vi "TLPM Measure Power2.vi"(8 "error in (no error)":errorcluster {"code" format="%.0x"}, 11 "instrument handle":refnum<visa-resource-name>) -> (0 "error out":errorcluster {"code" format="%.0x"}, 2 "Power":dbl, 3 "instrument handle out":refnum<visa-resource-name>)   [LabVIEW 2023, in "Thorlabs Power Meter.lvlib"]
doc: "This VI is used to obtain power readings from the instrument. \n\nRemark:\nThis VI starts a new measurement cycle and after finishing measurement the result is received. Subject to the actual Average Count this may take up to seconds. Refer to <Set/Get Average Count>."
uses:
  Thorlabs Power Meter.lvlib
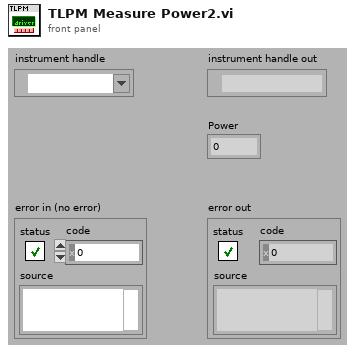
[diagram p1: front panel]
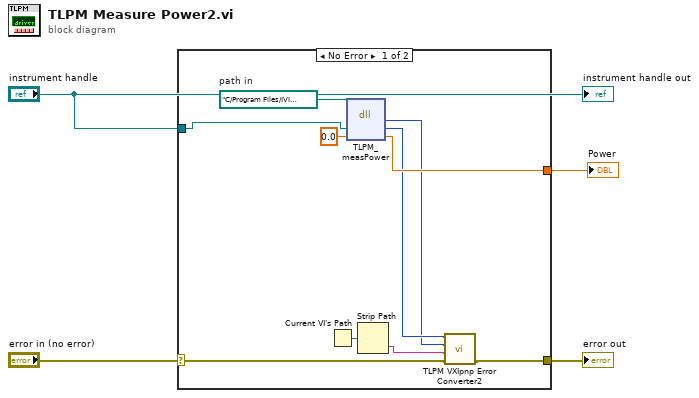
[diagram p0: block diagram]
diagram:
  n1 = case shown="No Error" "error in (no error)" {
    selector: "error in (no error)" -> [w9 w15]
    tunnel: [w10 w15] -> w4
    tunnel: "instrument handle" -> [w13 _]
    tunnel: [w11 _] -> w1
    frame No Error {
      w5 = path "C:/Program Files/IVI Foundation/VISA/Win64/Bin/TLPM_64.dll"  # path in
      n2 = Current VI's Path() -> (path=w14:path)
      n3 = dll-call lib="TLPM_64.dll" fn="TLPM_measPower"(path in=w5, "Instrument Handle"=w13, "Power"=0.0) -> ("return type"=w6:i32, "Instrument Handle"=w7:u32, "Power"=w11:dbl)  [unwired: 2 in, 2 out]
      n4 = Strip Path(path=w14) -> (name=w8:string)  [unwired: 1 out]
      n5 = call "TLPM VXIpnp Error Converter2.vi"("error in (no error)"=w9, "Name Of VI (\"\")"=w8, "CVI Error Code (0)"=w6, "instrument handle"=w7) -> ("error out"=w10:errorcluster)  [unwired: 6 in, 1 out]
    }
    frame Error {
    }
  }
  "error out" <- w4
  "Power" <- w1
  "instrument handle out" <- "instrument handle"
